vi "getIterator.vi"(8 "error in (no error)":errorcluster, 11 "NameRepository in":refnum<class "NameRepository.lvclass">) -> (0 "error out":errorcluster, 2 "NameIterator.lvclass":refnum<class "NameIterator.lvclass">, 3 "NameRepository out":refnum<class "NameRepository.lvclass">)   [LabVIEW 2018, in "NameRepository.lvclass"]
uses:
  NameRepository.lvclass
  NameIterator Class/NameIterator.lvclass
  NameRepository.lvclass/NameRepository.ctl
  NameIterator Class/NameIterator.lvclass/NameIterator.ctl
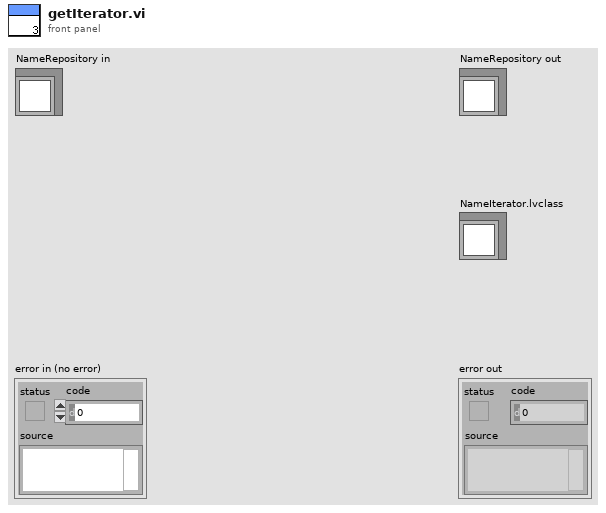
[diagram p1: front panel]
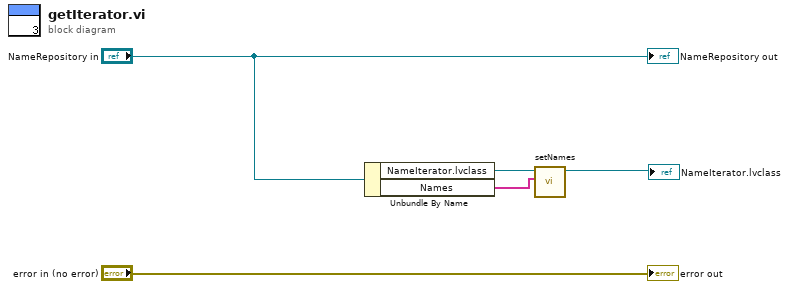
[diagram p0: block diagram]
diagram:
  n1 = Unbundle By Name("NameRepository in") -> ("NameIterator.lvclass"=w3:refnum<class "NameIterator.lvclass">, "Names"=w1:string[])
  n2 = call "setNames.vi"("Names"=w1, "NameIterator in"=w3) -> ("NameIterator out"=→"NameIterator.lvclass":refnum<class "NameIterator.lvclass">)  [unwired: 8 in, 1 out]
  "error out" <- "error in (no error)"
  "NameRepository out" <- "NameRepository in"
